vi "Launcher_Process Actor.vi"() -> ()   [LabVIEW 2022 SP3]
uses:
  Recipe View/Recipe View.lvclass
  XY Stage/Process Actor/View/XY Stage Class/XY Stage Class.lvclass
  C:/XY Stage/iView/base view/base view.lvclass
  Laser/Laser View/Laser View.lvclass
  IO Monitor/Class 3/DAQ View.lvclass
  Camera/Camera View/Camera View.lvclass
  IO Monitor/DAQ Controller/DAQ Controller.lvclass
  C:/XY Stage/IO Monitor/DAQ API/DAQ API.lvclass
  Laser/Laser Controller/Laser Controller.lvclass
  C:/XY Stage/Laser/Laser Controller api/Laser API.lvclass
  XY Stage/Process Actor/XY Controller/XY Stage Controller/XY Stage Controller.lvclass
  C:/XY Stage/XY Stage/Interfaces/2-Axis Stage API/2-Axis Stage Async API.lvclass
  Recipe Controller/Recipe Controller.lvclass
  C:/XY Stage/Process Actor Project/Recipe API/Recipe API.lvclass
  Recipe View/Accessors/Write Recipe API.lvclass.vi
  Recipe View/Accessors/Write Camera VIEW.vi
  Recipe View/Accessors/Write DAQ VIEW.vi
  Recipe View/Accessors/Write Laser VIEW.vi
  Recipe View/Accessors/Write XY stage VIEW.vi
  Camera/Camera Controller/Camera Controller.lvclass
  C:/XY Stage/XY Stage/Interfaces/2-Axis Async Home/2-Axis Async Home.lvclass
  C:/XY Stage/XY Stage/Interfaces/2-Axis Stage/2-Axis Stage Actions.lvclass
  C:/XY Stage/XY Stage/Interfaces/2-Axis Stage Status/2-Axis Stage Status.lvclass
  C:/XY Stage/XY Stage/Interfaces/Async Coms/Async Coms.lvclass
  C:/XY Stage/XY Stage/Process Actor/XY Controller/XY Stage Controller/XY Stage Controller.lvclass
  C:/XY Stage/Laser/Get Laser Status/Get Laser Status.lvclass
  C:/XY Stage/Laser/Laser API/Laser.lvclass
  C:/XY Stage/Laser/Laser Controller/Laser Controller.lvclass
  C:/XY Stage/IO Monitor/Aquire Data/Aquire Data.lvclass
  C:/XY Stage/IO Monitor/Get Daq Status/Get Daq Status.lvclass
  C:/XY Stage/IO Monitor/DAQ Controller/DAQ Controller.lvclass
  C:/XY Stage/Process Actor Project/Recipe/Recipe.lvclass
  C:/XY Stage/Process Actor Project/Recipe Status/Recipe Status.lvclass
  C:/XY Stage/Process Actor Project/Recipe Controller/Recipe Controller.lvclass
  C:/XY Stage/iView/iView/iView.lvclass
  C:/XY Stage/Camera/Camera View/Camera View.lvclass
  C:/XY Stage/IO Monitor/Class 3/DAQ View.lvclass
  C:/XY Stage/Laser/Laser View/Laser View.lvclass
  C:/XY Stage/XY Stage/Process Actor/View/XY Stage Class/XY Stage Class.lvclass
  C:/XY Stage/Camera/Camera Controller/Camera Controller.lvclass
  C:/XY Stage/Camera/Camera API/Camera API.lvclass
  C:/XY Stage/Camera/Camera Async Coms/Camera Async Coms.lvclass
panel:
  out "error out":errorcluster
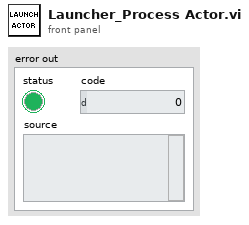
[diagram p1: front panel]
types:
  T1 = typedef "Recipe Comps.ctl" = cluster{"Laser View":refnum<class "Laser View.lvclass">, "Laser Controller ":refnum<class "Laser Controller.lvclass">, "Camera Controller":refnum<class "Camera Controller.lvclass">, "Camera View":refnum<class "Camera View.lvclass">, "DAQ Controller":refnum<class "DAQ Controller.lvclass">, "DAQ VIEW":refnum<class "DAQ View.lvclass">, "XY VIEW":refnum<class "XY Stage Class.lvclass">, "XY Stage Controller":refnum<class "XY Stage Controller.lvclass">}
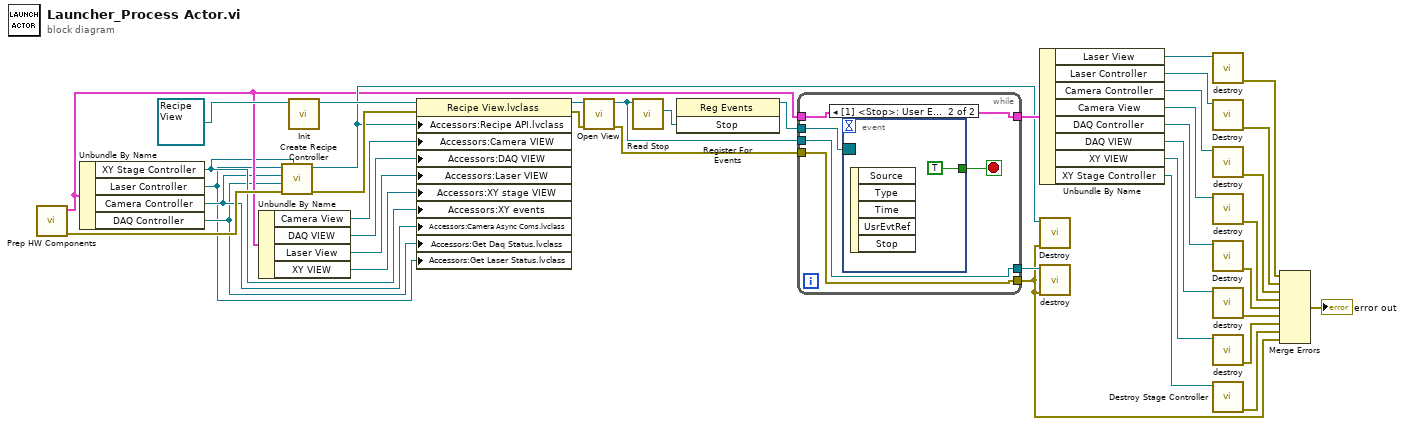
[diagram p0: block diagram]
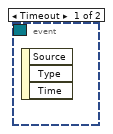
[diagram p2: hidden frame]
diagram:
  n1 = call "Prep HW Components.vi"() -> ("error out"=w22:errorcluster, "Recipe Comps"=w12:T1)  [unwired: 10 in]
  n2 = Unbundle By Name(w12) -> ("XY Stage Controller"=w4:refnum<class "XY Stage Controller.lvclass">, "Laser Controller"=w1:refnum<class "Laser Controller.lvclass">, "Camera Controller"=w3:refnum<class "Camera Controller.lvclass">, "DAQ Controller"=w2:refnum<class "DAQ Controller.lvclass">)
  n3 = Unbundle By Name(w12) -> ("Camera View"=w11:refnum<class "Camera View.lvclass">, "DAQ VIEW"=w10:refnum<class "DAQ View.lvclass">, "Laser View"=w9:refnum<class "Laser View.lvclass">, "XY VIEW"=w8:refnum<class "XY Stage Class.lvclass">)
  n4 = call "Create Recipe Controller.vi"("2-Axis Stage Async API.lvclass"=w4, "error in (no error)"=w22, "DAQ API.lvclass"=w2, "Camera Controller"=w3, "Laser API.lvclass"=w1) -> ("error out"=w20:errorcluster, "Recipe Controller.lvclass"=w13:refnum<class "Recipe Controller.lvclass">)  [unwired: 5 in]
  n5 = call-dynamic "Init.vi"("Recipe View in"=refnum<class "Recipe View.lvclass"> refnum ("Recipe View.lvclass")) -> ("Recipe View out"=w15:refnum<class "Recipe View.lvclass">)  [unwired: 9 in, 1 out]
  n6 = property class="Recipe View.lvclass"(reference=w15, error in=w20, "Accessors:Recipe API.lvclass"=w13, "Accessors:Camera VIEW"=w11, "Accessors:DAQ VIEW"=w10, "Accessors:Laser VIEW"=w9, "Accessors:XY stage VIEW"=w8, "Accessors:XY events"=w4, "Accessors:Camera Async Coms.lvclass"=w3, "Accessors:Get Daq Status.lvclass"=w2, "Accessors:Get Laser Status.lvclass"=w1) -> (reference out=w14:refnum<class "Recipe View.lvclass">, error out=w16:errorcluster)
  n7 = call-dynamic "Open View.vi"("error in (no error)"=w16, "base view in"=w14) -> ("error out"=w19:errorcluster, "base view out"=w7:refnum<class "Recipe View.lvclass">)  [unwired: 8 in]
  n8 = call "Read Stop.vi"("In"=w7) -> ("Stop"=w6:refnum<user-event>)  [unwired: 8 in, 2 out]
  n9 = register-events(w6) -> (reference out=w5:refnum<event-registration>)  [unwired: 2 in, 1 out]
  n10 = while {
    tunnel: w12 -> [w45]
    tunnel: [w45] -> w40
    tunnel: w19 -> [w43]
    tunnel: [w43] -> w17
    tunnel: w7 -> [w42]
    tunnel: [w42] -> w18
    tunnel: w5 -> [w41]
    stop <- w44 stop-if-true
    n11 = event shown="[1] <Stop>: User Event" {
      selector: w41 -> [_ _]
      dyn-events: _ -> [_ _]
      timeout: _ -> [_ _]
      tunnel: [_ TRUE] -> w44
      event Timeout {
        n12 = event-data() -> ()  [unwired: 1 in, 3 out]
      }
      event User Event {
        n13 = event-data() -> ()  [unwired: 1 in, 5 out]
      }
    }
  }
  n14 = Unbundle By Name(w40) -> ("Laser View"=w32:refnum<class "Laser View.lvclass">, "Laser Controller"=w33:refnum<class "Laser Controller.lvclass">, "Camera Controller"=w34:refnum<class "Camera Controller.lvclass">, "Camera View"=w35:refnum<class "Camera View.lvclass">, "DAQ Controller"=w36:refnum<class "DAQ Controller.lvclass">, "DAQ VIEW"=w37:refnum<class "DAQ View.lvclass">, "XY VIEW"=w39:refnum<class "XY Stage Class.lvclass">, "XY Stage Controller"=w38:refnum<class "XY Stage Controller.lvclass">)
  n15 = call-dynamic "Destroy.vi"("error in (no error)"=w17, "Recipe Controller in"=w13) -> ()  [unwired: 8 in, 2 out]
  n16 = call-dynamic "destroy.vi"("error in (no error)"=w17, "base view in"=w18) -> ()  [unwired: 8 in, 2 out]
  n17 = call-dynamic "destroy.vi"("Laser View in"=w32) -> ("error out"=w31:errorcluster)  [unwired: 9 in, 1 out]
  n18 = call "Destroy.vi"("Laser Controller in"=w33) -> ("error out"=w30:errorcluster)  [unwired: 9 in, 1 out]
  n19 = call-dynamic "destroy.vi"("Camera Controller in"=w34) -> ("error out"=w29:errorcluster)  [unwired: 9 in, 1 out]
  n20 = call-dynamic "destroy.vi"("Camera View in"=w35) -> ("error out"=w28:errorcluster)  [unwired: 9 in, 1 out]
  n21 = call "Destroy.vi"("DAQ Controller in"=w36) -> ("error out"=w27:errorcluster)  [unwired: 9 in, 1 out]
  n22 = call-dynamic "destroy.vi"("DAQ View in"=w37) -> ("error out"=w26:errorcluster)  [unwired: 9 in, 1 out]
  n23 = call-dynamic "destroy.vi"("XY Stage Class in"=w39) -> ("error out"=w25:errorcluster)  [unwired: 9 in, 1 out]
  n24 = call "Destroy Stage Controller.vi"("XY Stage Controller in"=w38) -> ("error out"=w24:errorcluster)  [unwired: 9 in, 1 out]
  n25 = Merge Errors(w31, w30, w29, w28, w27, w26, w25, w24, w17) -> (→"error out":errorcluster)
